vi "setInputPathReplacement.vi"(8 "error in (no error)":errorcluster, 10 "replacementPattern":path, 11 "VGS_Job in":refnum<class "VGS_Job.lvclass">) -> (0 "error out":errorcluster, 3 "VGS_Job out":refnum<class "VGS_Job.lvclass">)   [LabVIEW 2022 SP3, in "LV_VGS.lvlib" / "VGS_Job.lvclass"]
uses:
  VGS_Job.lvclass
  VGS_Job.lvclass/VGS_Job.ctl
  C:/Users/Andrey/Documents/GitHub/LV_VGS/vgs_project.dll
  vgs_project.dll
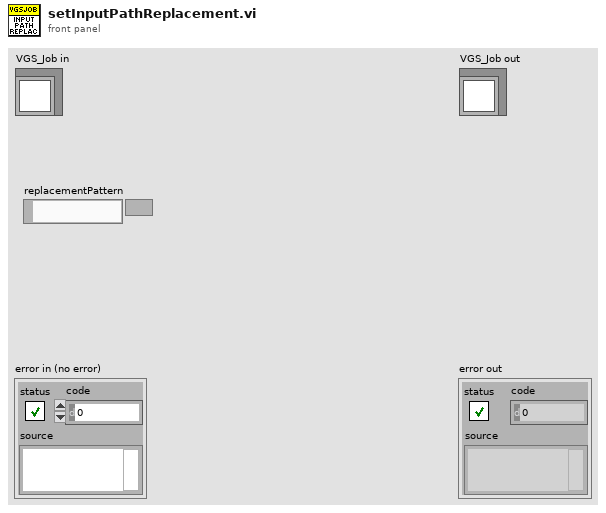
[diagram p1: front panel]
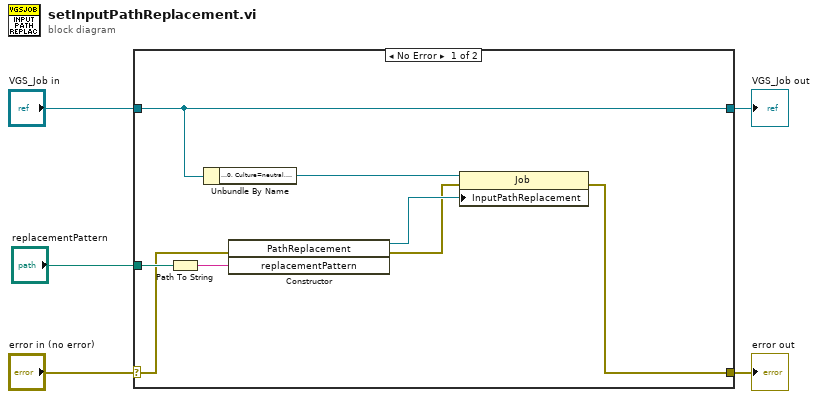
[diagram p0: block diagram]
diagram:
  n1 = case shown="No Error" "error in (no error)" {
    selector: "error in (no error)" -> [w9 w15]
    tunnel: [w7 w15] -> w4
    tunnel: [w13 w14] -> w2
    tunnel: "VGS_Job in" -> [w13 w14]
    tunnel: "replacementPattern" -> [w10 _]
    frame No Error {
      n2 = Path To String(path=w10) -> (string=w6:string)
      n3 = Unbundle By Name(w13) -> ("Job reference"=w12:refnum<k24>)
      n4 = constructor class="Job+PathReplacement"(error in=w9, "replacementPattern"=w6) -> (reference out=w11:refnum<k24>, error out=w8:errorcluster)  [unwired: 2 in, 2 out]
      n5 = property class="Job"(reference=w12, error in=w8, "InputPathReplacement"=w11) -> (error out=w7:errorcluster)  [unwired: 1 out]
    }
    frame Error {
    }
  }
  "error out" <- w4
  "VGS_Job out" <- w2
